vi "TstBldr_Project.vi"(0 "Engine reference":refnum<k7>, 1 "Condition run?":bool, 3 "Paths":T1, 5 "Sequence File Ref":refnum<k7>, 7 "VeriStand version info":T2, 9 "Project Name":string="Open Workspace Manager Reference", 11 "error in":errorcluster, 12 "Requirement":string, 13 "Sequence index":i32, 14 "Attended?":bool) -> (4 "Engine reference (out)":refnum<k7>, 6 "Sequence File Ref(out)":refnum<k7>, 10 "Sequence index out":i32, 15 "error out":errorcluster)   [LabVIEW 2010]
doc: "This VI creates the TestStand steps to:\n- Open a VeriStand Project Reference\n- Open the Workspace (if attended execution is selected)\n- Deploy system configuration and connect"
uses:
  SeqBuilder/Ctls/dotNetAssemblyInfo.ctl
  SeqBuilder/Ctls/VSModuleTokens.ctl
  FilePaths.ctl
  vs_RunWorkspaceSteps.ctl
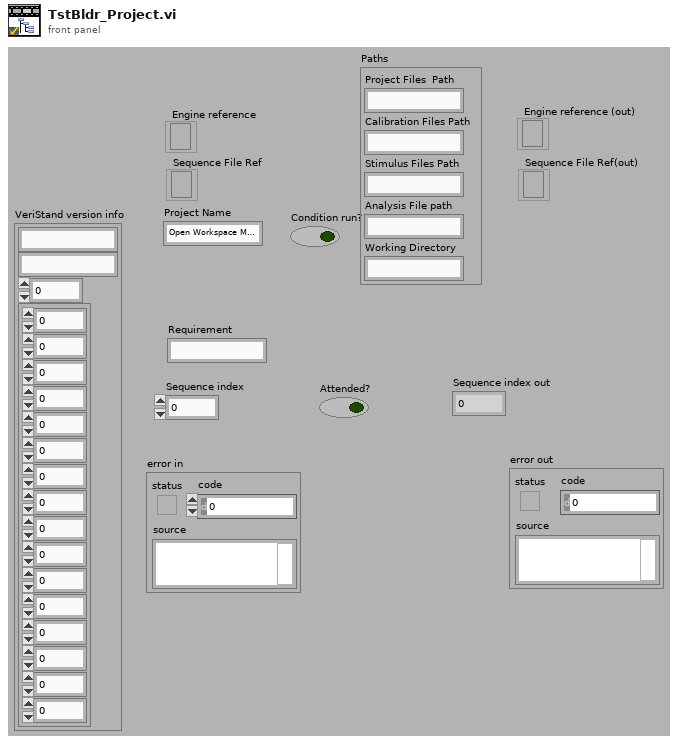
[diagram p1: front panel]
types:
  T1 = typedef "FilePaths.ctl" = cluster{"Project Files  Path":string, "Calibration Files Path":string, "Stimulus Files Path":string, "Analysis File path":string, "Working Directory":string}
  T2 = typedef "dotNetAssemblyInfo.ctl" = cluster{"VeriStand.exe Path":string, "Assembly":string, "Constructor Token":i32, "Module Token":T3}
  T3 = typedef "VSModuleTokens.ctl" = cluster{"GetIWorkspaceToken":i32, "GetIStimulusToken":i32, "GetIModelManagerToken":i32, "GetIProjectToken":i32, "RunProjectToken":i32, "CloseProjectToken":i32, "RunWorkspaceToken":i32, "StopWorkspaceToken":i32, "SetSingleChannelToken":i32, "SetMultipleParametersToken":i32, "RunStimulusToken":i32, "GetStimulusStateToken":i32, "Open WorkspaceToken":i32, "DeployToken":i32, "UndeployToken":i32, "QuitToken":i32}
  T4 = typedef "vs_RunWorkspaceSteps.ctl" = enum16{"Open Project", "Open Workspace", "Deploy and Connect", "Exit loop"}
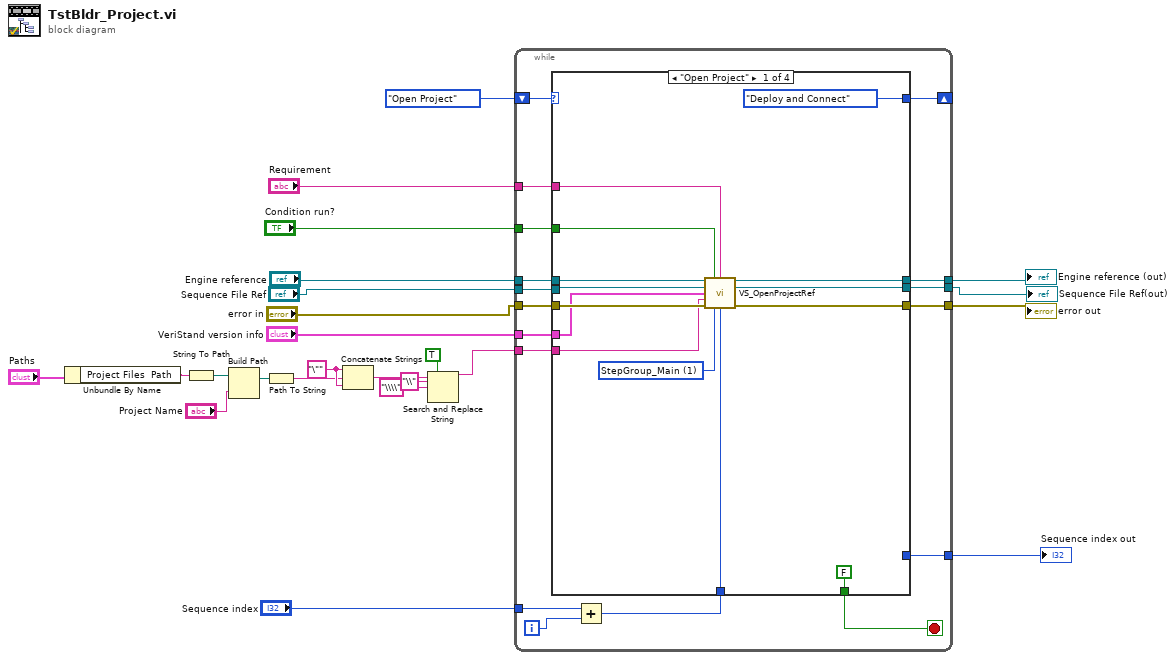
[diagram p0: block diagram]
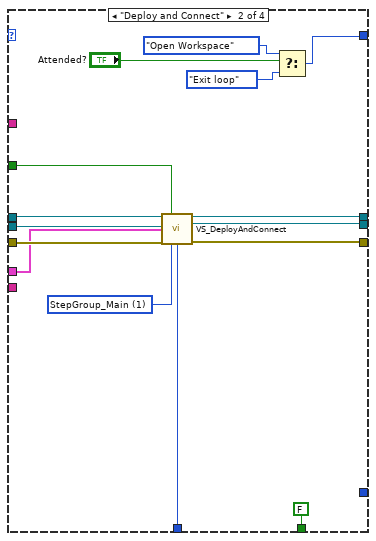
[diagram p2: hidden frame]
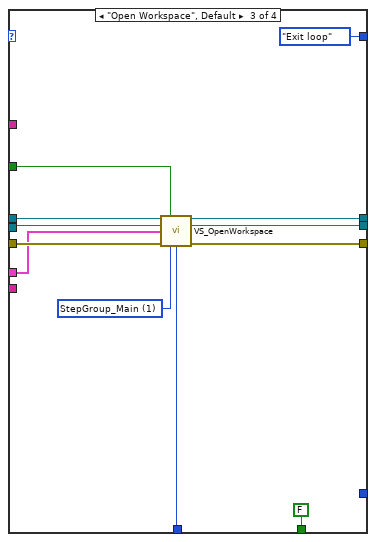
[diagram p3: hidden frame]
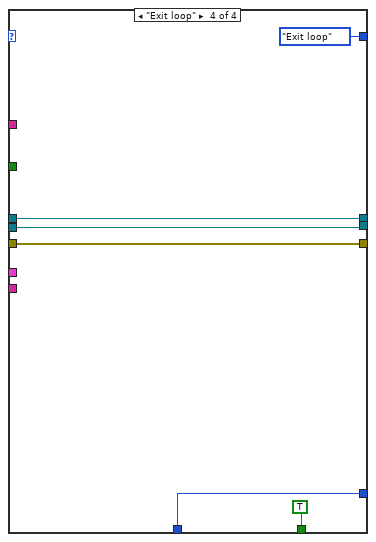
[diagram p4: hidden frame]
diagram:
  w14 = "\"" ("string")
  n1 = Unbundle By Name("Paths") -> ("Project Files  Path"=w2:string)
  n2 = String To Path(string=w2) -> (path=w1:path)
  n3 = Build Path(base path=w1, name or relative path="Project Name") -> (appended path=w9:path)
  n4 = Path To String(path=w9) -> (string=w7:string)
  n5 = Concatenate Strings(w14, w7, w14) -> (w10:string)
  n6 = Search and Replace String(replace all?=TRUE ("replace all? (F)"), input string=w10, search string="\\", replace string="\\\\" ("replace string (\"\")")) -> (result string=w6:string)  [unwired: 4 in, 3 out]
  n7 = while {
    shift-right: [w40] -> _
    shift-left: vs_RunWorkspaceSteps."Open Project" ("Enum") -> [w41]
    tunnel: "Engine reference" -> [w39]
    tunnel: "error in" -> [w38]
    tunnel: [w37] -> w21
    tunnel: [w36] -> w20
    tunnel: "Sequence index" -> [w35]
    tunnel: "Sequence File Ref" -> [w32]
    tunnel: "VeriStand version info" -> [w31]
    tunnel: "Condition run?" -> [w29]
    tunnel: w6 -> [w28]
    tunnel: "Requirement" -> [w27]
    tunnel: [w26] -> w5
    tunnel: [w25] -> w4
    i -> [w34]
    stop <- w30 stop-if-true
    n8 = Add(x=w35, y=w34) -> (x+y=w33:i32)
    n9 = case shown="\"Open Project\"" w41 {
      tunnel: [vs_RunWorkspaceSteps."Deploy and Connect" ("Enum") w57 vs_RunWorkspaceSteps."Exit loop" ("Enum") vs_RunWorkspaceSteps."Exit loop" ("Enum")] -> w40
      tunnel: w39 -> [w55 w64 w78 w87]
      tunnel: w38 -> [w54 w69 w80 w86]
      tunnel: [w53 w66 w77 w87] -> w37
      tunnel: [w52 w68 w79 w86] -> w36
      tunnel: w33 -> [w51 w67 w72 w83]
      tunnel: w32 -> [w49 w63 w76 w84]
      tunnel: w31 -> [w48 w61 w74 _]
      tunnel: [FALSE ("stop") FALSE ("stop") FALSE ("stop") TRUE ("stop")] -> w30
      tunnel: w29 -> [w47 w62 w73 _]
      tunnel: w28 -> [w46 _ _ _]
      tunnel: w27 -> [w45 _ _ _]
      tunnel: [w43 w65 w75 w84] -> w26
      tunnel: [_ _ _ w83] -> w25
      frame "Open Project" {
        w50 = 1 items=["StepGroup_Setup", "StepGroup_Main", "StepGroup_Cleanup"] ("Step Group")
        n10 = call "VS_OpenProjectRef.vi"("Engine Reference(in)"=w55, "Condition Run?"=w47, "Requirement"=w45, "Sequence File Ref(in)"=w49, "VeriStand version info"=w48, "Project path"=w46, "error in"=w54, "Step Group"=w50, "Step Index"=w51) -> ("Engine reference(out)"=w53:refnum<k7>, "Sequence File Ref(out)"=w43:refnum<k7>, "error out"=w52:errorcluster)  [unwired: 3 in, 1 out]
      }
      frame "Deploy and Connect" {
        w60 = 1 items=["StepGroup_Setup", "StepGroup_Main", "StepGroup_Cleanup"] ("Step Group")
        n11 = call "VS_DeployAndConnect.vi"("Engine Reference(in)"=w64, "Condition Run?"=w62, "Sequence File Ref(in)"=w63, "VeriStand version info"=w61, "error in"=w69, "Step Group"=w60, "Step Index"=w67) -> ("Engine reference(out)"=w66:refnum<k7>, "Sequence File Ref(out)"=w65:refnum<k7>, "error out"=w68:errorcluster)  [unwired: 5 in, 1 out]
        n12 = Select(t=vs_RunWorkspaceSteps."Open Workspace" ("Enum"), s="Attended?", f=vs_RunWorkspaceSteps."Exit loop" ("Enum")) -> (s? t:f=w57:T4)
      }
      frame "Open Workspace", Default {
        w71 = 1 items=["StepGroup_Setup", "StepGroup_Main", "StepGroup_Cleanup"] ("Step Group")
        n13 = call "VS_OpenWorkspace.vi"("Engine Reference(in)"=w78, "Condition Run?"=w73, "Sequence File Ref(in)"=w76, "VeriStand version info"=w74, "error in"=w80, "Step Group"=w71, "Step Index"=w72) -> ("Engine reference(out)"=w77:refnum<k7>, "Sequence File Ref(out)"=w75:refnum<k7>, "error out"=w79:errorcluster)  [unwired: 5 in, 1 out]
      }
      frame "Exit loop" {
      }
    }
  }
  "error out" <- w20
  "Sequence File Ref(out)" <- w5
  "Engine reference (out)" <- w21
  "Sequence index out" <- w4
